vi "Read Info from File.vi"(8 "error in (no error)":errorcluster, 11 "LabVIEW File in":refnum<class "LabVIEW File.lvclass">) -> (0 "error out":errorcluster, 3 "LabVIEW File out":refnum<class "LabVIEW File.lvclass">)   [LabVIEW 2020, in "Save for Previous Version.lvlib" / "LabVIEW File.lvclass"]
uses:
  LabVIEW File.lvclass
  File/File.lvclass/File.lvclass
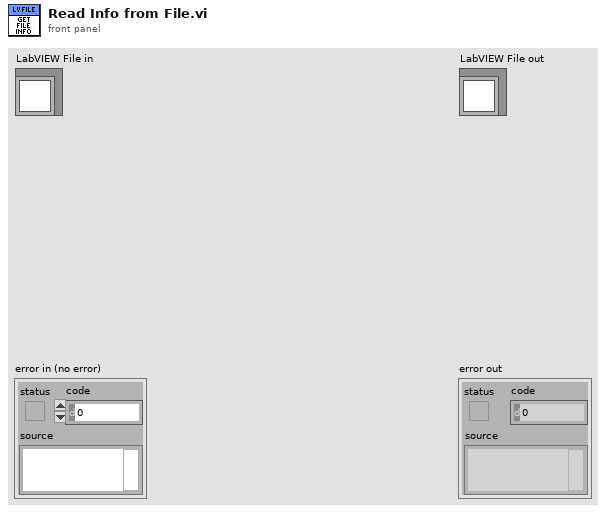
[diagram p1: front panel]
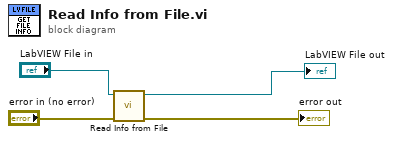
[diagram p0: block diagram]
diagram:
  n1 = call-parent "Read Info from File.vi"("error in (no error)"="error in (no error)", "File in"="LabVIEW File in") -> ("error out"=→"error out":errorcluster, "File out"=→"LabVIEW File out":refnum<class "LabVIEW File.lvclass">)  [unwired: 8 in]
